vi "HGF_SVMonitor.appendData2Variant.vi"(2 "timeout in ms(10)":i32=10, 3 "error in (no error)":errorcluster, 4 "initData":variant) -> (0 "error out":errorcluster, 1 "dup initData":variant)   [LabVIEW 2012, in "HGF_SV.lvlib" / "HGF_SVMonitor.lvclass"]
uses:
  HGF_SVMonitor.lvclass
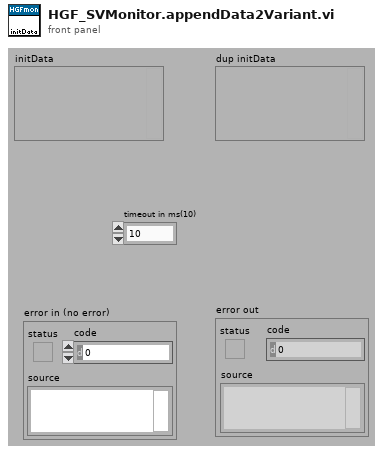
[diagram p1: front panel]
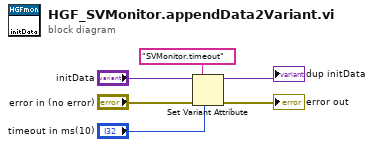
[diagram p0: block diagram]
diagram:
  n1 = Set Variant Attribute(Variant="initData", name="SVMonitor.timeout", value="timeout in ms(10)", error in="error in (no error)") -> (Variant out=→"dup initData":variant, error out=→"error out":errorcluster)  [unwired: 1 out]
